vi "Single-process Shared Variable Method.vi"() -> ()   [LabVIEW 2015]
uses:
  <vilib>/platform/TimedLoop/XDataNode/XDataNode.xnode
  <vilib>/Platform/TimedLoop/XDataNode/nitl_modes.ctl
  <vilib>/Platform/TimedLoop/XDataNode/XDNodeRunTimeDep.lvlib
  <vilib>/Platform/TimedLoop/XDataNode/wakeup.ctl
  <vilib>/Platform/TimedLoop/XDataNode/timing_clust.ctl
panel:
  out "Overflow":bool
  out "Result Data":dbl(graph)
  in  "Waveform Type":T1(ring)
  in  "Amplitude":dbl(knob)=1.0 scale=0.0..1.0 scale format="%.1f"
  in  "Stop":bool
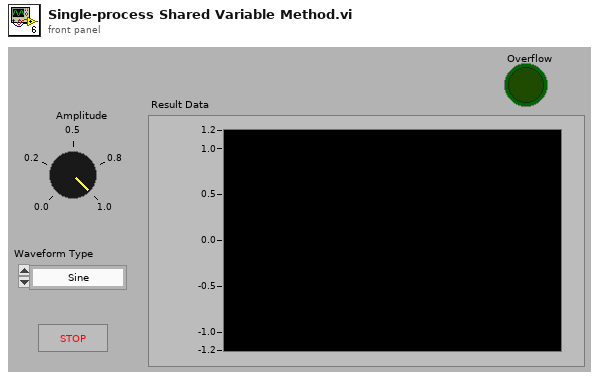
[diagram p1: front panel]
types:
  T1 = enum16{"Sine", "Square", "Triangle", "Random Noise"}
  T2 = typedef "XDNodeRunTimeDep.lvlib/timing_clust.ctl" = cluster{"Expected End [f-1]":u64, "Actual End [f-1]":u64, "Finished Late? [f-1]":bool, "Expected End [i-1]":u64, "Actual End [i-1]":u64, "Finished Late? [i-1]":bool, "Expected Start [i]":u64, "Actual Start [i]":u64, "Expected Start [f]":u64, "Actual Start [f]":u64, "Source Name":string, "Structure Name":string, "Period":i64, "Deadline":i64, "Offset":i64, "Start":i64, "Priority":i32, "Timeout":i32, "Mode":T3, "Wakeup Reason":T4, "Error":errorcluster, "Source Type":string, "Secondary Source Type":string, "Global End Time":u64, "Global Start Time":u64, "Frame Duration":u64, "Iteration Duration":u64, "Assigned CPU":i32, "I/O Scan Engine Mode":u32}
  T3 = typedef "XDNodeRunTimeDep.lvlib/nitl_modes.ctl" = enum32{"No Change", "Process missed periods, maintain original phase", "Discard missed periods, maintain original phase", "Process missed periods, ignore original phase", "Discard missed periods, ignore original phase"}
  T4 = typedef "XDNodeRunTimeDep.lvlib/wakeup.ctl" = enum32{"Normal", "Aborted", "Asynchronous wakeup", "Timing source error", "Timed loop error", "Timeout"}
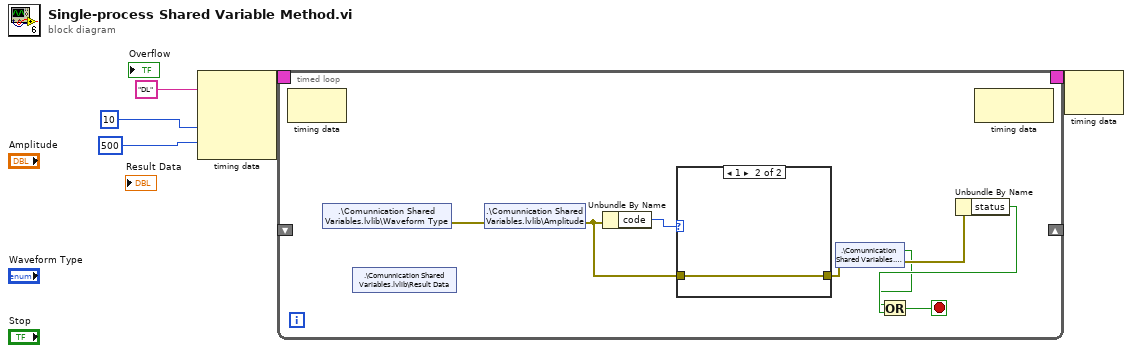
[diagram p0: block diagram]
diagram:
  n1 = node-c288("DL" ("Structure Name"), i64 10 ("Period"), 500 ("Priority")) -> (w5:T2)  [unwired: 1 in]
  n2 = timed-loop {
    timing: w5 -> [_]
    timing-out: [_] -> w4
    shift-right: _ -> [_]
    shift-left: _ -> [_]
    stop <- w8 stop-if-true
    n3 = node-c288() -> ()  [unwired: 1 in, 1 out]
    n4 = shared-variable ".\\Comunnication Shared Variables.lvlib\\Waveform Type"() -> (error out=w13:errorcluster)  [unwired: 1 in, 1 out]
    n5 = shared-variable ".\\Comunnication Shared Variables.lvlib\\Result Data"() -> ()  [unwired: 2 in, 1 out]
    n6 = shared-variable ".\\Comunnication Shared Variables.lvlib\\Amplitude"(error in=w13) -> (error out=w11:errorcluster)  [unwired: 1 out]
    n7 = Unbundle By Name(w11) -> ("code"=w12:i32)
    n8 = case shown="1" w12 {
      tunnel: w11 -> [_ w14]
      tunnel: [_ w14] -> w10
      frame 0, Default {
      }
      frame 1 {
      }
    }
    n9 = shared-variable ".\\Comunnication Shared Variables.lvlib\\Stop"(error in=w10) -> (w6:bool, error out=w9:errorcluster)
    n10 = Unbundle By Name(w9) -> ("status"=w7:bool)
    n11 = Or(x=w6, y=w7) -> (x .or. y?=w8:bool)
    n12 = node-c288() -> ()  [unwired: 1 in, 1 out]
  }
  n13 = node-c288(w4) -> ()  [unwired: 1 out]
